vi "CCGetDICOMValuesToExcel.vi"(8 "error in (no error)":errorcluster, 11 "filename":string) -> (0 "error out":errorcluster, 2 "Values":string[](array[string]), 3 "itemTags":string[](array[string])=["PatientsName", "PatientId", "AccessionNumber", "ReferringPhysiciansName", "RequestingPhysician", "OperatorsName", "RequestedProcedureDescription", "RequestedProcedureId", "StudyInstanceUid", "StudyId", "SeriesInstanceUid"])   [LabVIEW 2013, in "main.lvlib" / "ClearCanvasLibrary.lvlib"]
uses:
  ClearCanvasLibrary.lvlib
  C:/Users/Simon/SkyDrive/LabView/2013/DM2020/DICOM/ClearCanvasNewBuild/ClearCanvas.Dicom.dll
  ClearCanvasNewBuild/ClearCanvas.Dicom.dll
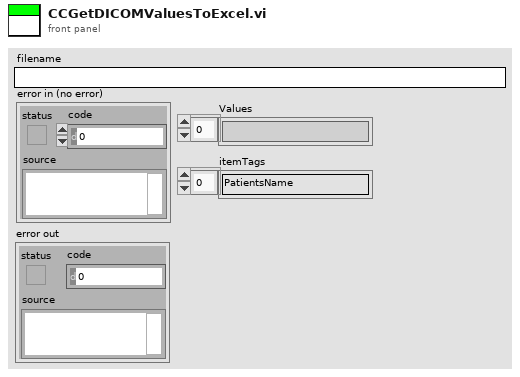
[diagram p1: front panel]
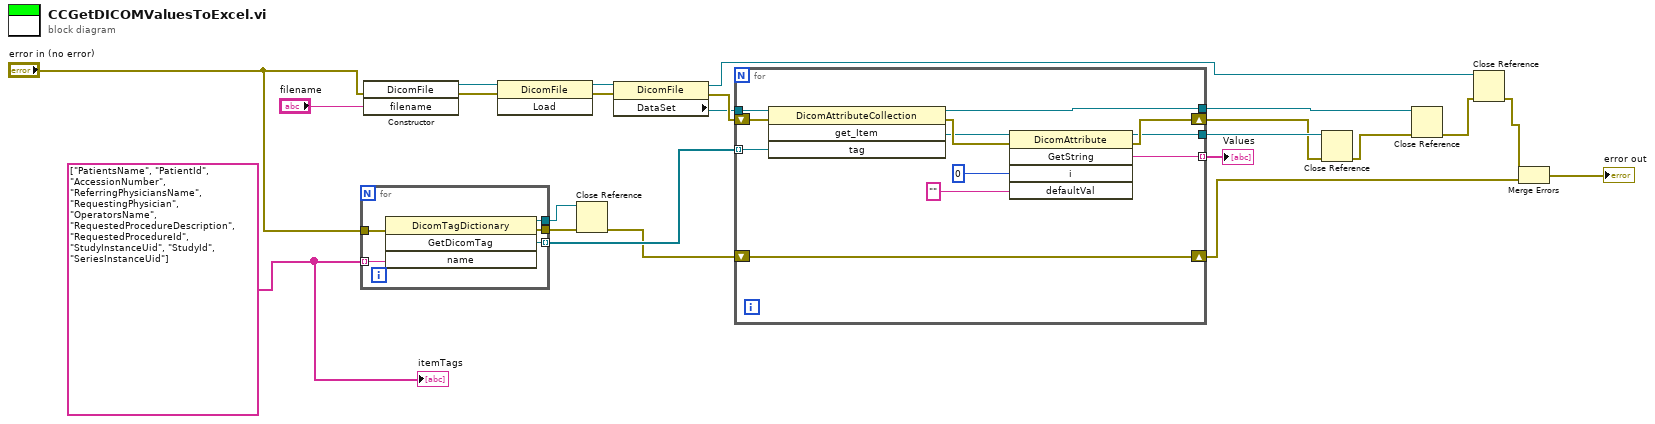
[diagram p0: block diagram]
diagram:
  w6 = string[] ["PatientsName", "PatientId", "AccessionNumber", "ReferringPhysiciansName", "RequestingPhysician", "OperatorsName", "RequestedProcedureDescription", "RequestedProcedureId", "StudyInstanceUid", "StudyId", "SeriesInstanceUid"]
  n1 = for {
    tunnel: "error in (no error)" -> [w28]
    tunnel: w6 -> [w27] mode=indexing
    tunnel: [w26] -> w7 mode=indexing
    tunnel: [w25] -> w4
    tunnel: [w24] -> w3
    n2 = invoke class="DicomTagDictionary" method="GetDicomTag"(error in=w28, "name"=w27) -> (reference out=w24:refnum<k24>, error out=w25:errorcluster, "GetDicomTag"=w26:refnum<k24>)  [unwired: 2 in, 1 out]
  }
  n3 = constructor class="DicomFile"(error in="error in (no error)", "filename"="filename") -> (reference out=w23:refnum<k24>, error out=w20:errorcluster)  [unwired: 2 in, 2 out]
  n4 = invoke class="DicomFile" method="Load"(reference=w23, error in=w20) -> (reference out=w21:refnum<k24>, error out=w19:errorcluster)  [unwired: 1 in, 1 out]
  n5 = Close Reference(reference=w3, error in (no error)=w4) -> (error out=w2:errorcluster)
  n6 = property class="DicomFile"(reference=w21, error in=w19) -> (reference out=w12:refnum<k24>, error out=w14:errorcluster, "DataSet"=w11:refnum<k24>)
  n7 = for {
    tunnel: w11 -> [w32]
    shift-right: [w35] -> w16
    shift-left: w14 -> [w40]
    tunnel: [w37] -> w18 mode=indexing
    tunnel: [w34] -> w17
    tunnel: [w30] -> w1
    tunnel: w7 -> [w33] mode=indexing
    shift-right: [w29] -> w10
    shift-left: w2 -> [w29]
    n8 = invoke class="DicomAttributeCollection" method="get_Item"(reference=w32, error in=w40, "tag"=w33) -> (reference out=w30:refnum<k24>, error out=w36:errorcluster, "get_Item"=w31:refnum<k24>)  [unwired: 1 in, 1 out]
    n9 = invoke class="DicomAttribute" method="GetString"(reference=w31, error in=w36, "i"=0, "defaultVal"="") -> (reference out=w34:refnum<k24>, error out=w35:errorcluster, "GetString"=w37:string)  [unwired: 1 in, 2 out]
  }
  "Values" <- w18
  n10 = Close Reference(reference=w17, error in (no error)=w16) -> (error out=w15:errorcluster)
  n11 = Close Reference(reference=w1, error in (no error)=w15) -> (error out=w13:errorcluster)
  n12 = Close Reference(reference=w12, error in (no error)=w13) -> (error out=w9:errorcluster)
  n13 = Merge Errors(w9, w10) -> (→"error out":errorcluster)
  "itemTags" <- w6
